vi "Draw Rectangle (ARGB).vi"(5 "Thickness (Default: 1)":i32=1, 6 "OpenCV Line Type (Default LINE_8)":T4=enum."LINE_8", 7 "ARGB Colour":T3={"Alpha"=255, "RGB"=0}, 8 "error in (no error)":errorcluster, 9 "Point B":T1, 10 "Point A":T1, 11 "ARGB Image":T2) -> (0 "error out":errorcluster, 3 "ARGB Image (Duplicate)":T2)   [LabVIEW 2020, in "g_ar_toolkit.image.lvlib"]
uses:
  g_ar_toolkit.image.lvlib
  Line Type.ctl
  g_ar_toolkit.common/Image Point (Integer).ctl
  ARGB Image.ctl
  ARGB Colour.ctl
  7e6fb015-3761-4366-a0a7-e436eb229083.vi
  g_ar_toolkit.common/Module Path.vi
  <vilib>/Utility/error.llb/Error Cluster From Error Code.vi
  g_ar_toolkit.common/g_ar_toolkit.common.lvlib
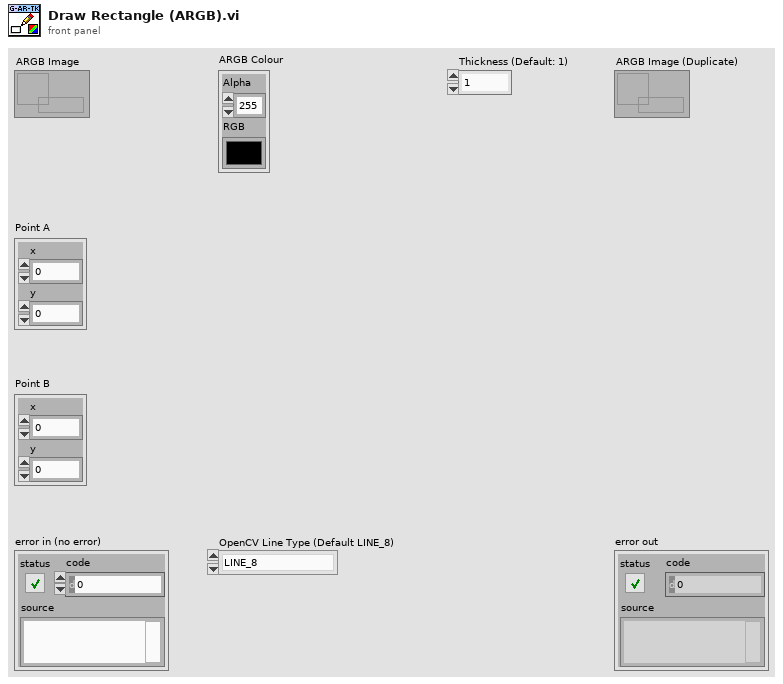
[diagram p1: front panel]
types:
  T1 = typedef "g_ar_toolkit.common.lvlib/Image Point (Integer).ctl" = cluster{"x":i32, "y":i32}
  T2 = typedef "g_ar_toolkit.image.lvlib/ARGB Image.ctl" = refnum<data-value>
  T3 = typedef "g_ar_toolkit.image.lvlib/ARGB Colour.ctl" = cluster{"Alpha":u8, "RGB":u32}
  T4 = typedef "g_ar_toolkit.image.lvlib/Line Type.ctl" = enum8{"FILLED", "LINE_4", "LINE_8", "LINE_AA"}
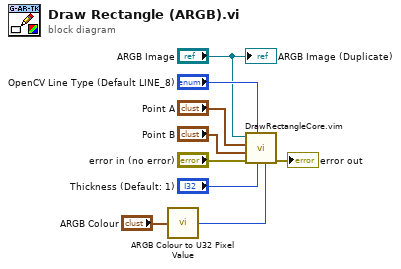
[diagram p0: block diagram]
diagram:
  n1 = call "ARGB Colour to U32 Pixel Value.vi"("ARGB Colour"="ARGB Colour") -> ("U32 Colour"=w3:u32)
  n2 = call "DrawRectangleCore.vim"("Colour"=w3, "Thickness"="Thickness (Default: 1)", "OpenCV Line Type"="OpenCV Line Type (Default LINE_8)", "error in (no error)"="error in (no error)", "Point B"="Point B", "Point A"="Point A", "Src"="ARGB Image") -> ("error out"=→"error out":errorcluster)  [unwired: 4 in]
  "ARGB Image (Duplicate)" <- "ARGB Image"
